vi "Sample To use2.vi"() -> ()   [LabVIEW 2014]
uses:
  Event_class/EventMsg.lvclass
panel:
  in  "Name":string
  out "Msg 3":string
  in  "stop":bool
  in  "Msg 2":string="q2333"
  out "Msg":string
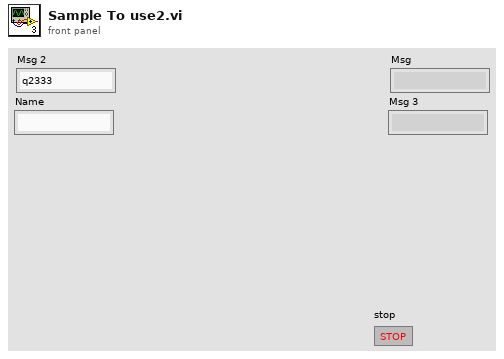
[diagram p1: front panel]
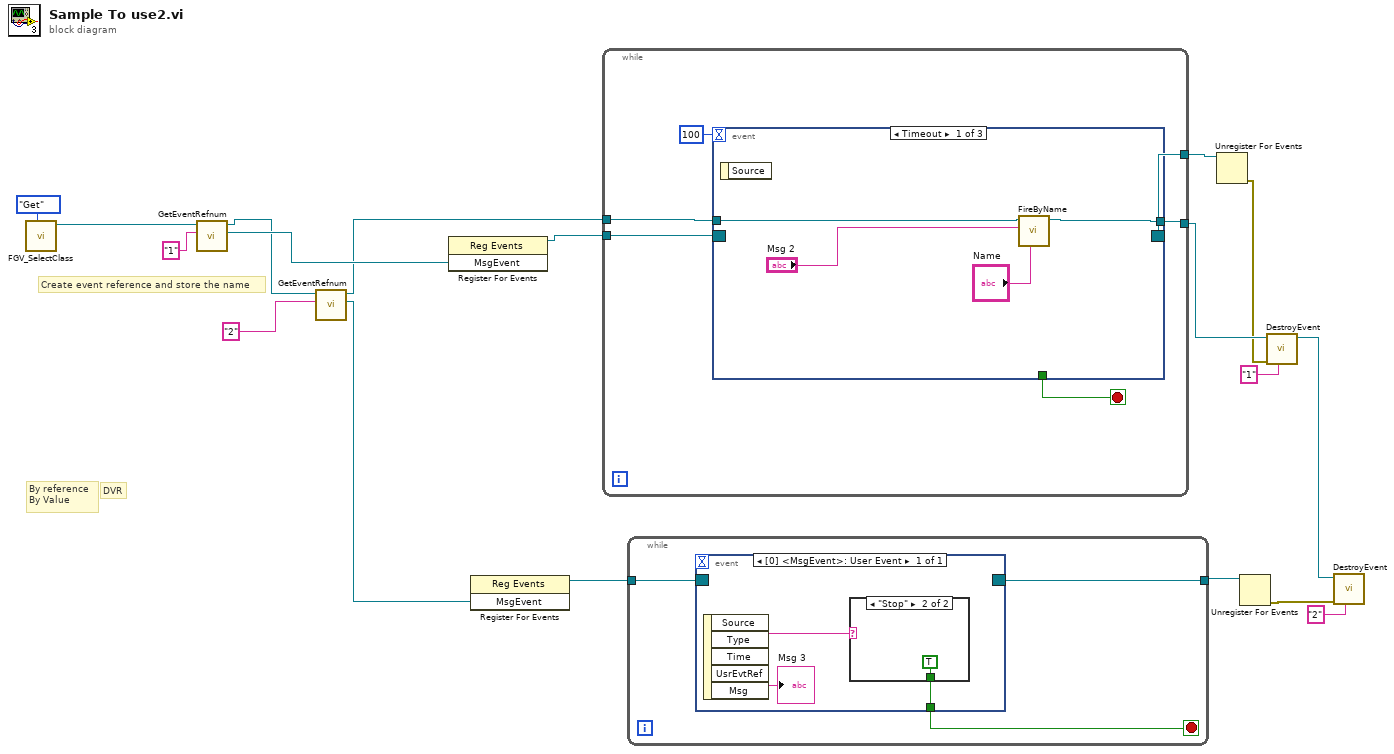
[diagram p0: block diagram]
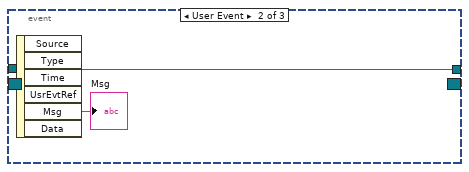
[diagram p3: hidden frame]
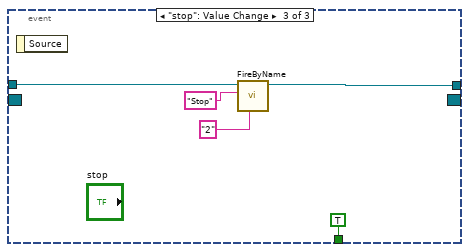
[diagram p4: hidden frame]
diagram:
  # "DVR"
  # "By reference \nBy Value"
  # "Create event reference and store the name"
  n1 = call "FGV_SelectClass.vi"("Action"=enum16{"Set", "Get"}."Get") -> ("EventMsg.lvclass 2"=w1:refnum<class "EventMsg.lvclass">)  [unwired: 10 in]
  n2 = call-dynamic "GetEventRefnum.vi"("Name"="1", "object in"=w1) -> ("MsgEvent"=w8:refnum<user-event>, "object out"=w6:refnum<class "EventMsg.lvclass">)  [unwired: 7 in, 1 out]
  n3 = call-dynamic "GetEventRefnum.vi"("Name"="2", "object in"=w6) -> ("MsgEvent"=w5:refnum<user-event>, "object out"=w3:refnum<class "EventMsg.lvclass">)  [unwired: 7 in, 1 out]
  n4 = register-events(w8) -> (reference out=w18:refnum<event-registration>)  [unwired: 2 in, 1 out]
  n5 = register-events(w5) -> (reference out=w17:refnum<event-registration>)  [unwired: 2 in, 1 out]
  n6 = while {
    tunnel: w18 -> [w23]
    tunnel: w3 -> [w21]
    tunnel: [w20] -> w15
    tunnel: [w19] -> w14
    stop <- w24 stop-if-true
    n7 = event shown="[0] Timeout" {
      selector: w23 -> [_ _ _]
      dyn-events: [_ _ _] -> w19
      timeout: 100 -> [_ _ _]
      tunnel: w21 -> [w27 w29 w33]
      tunnel: [_ _ TRUE ("stop")] -> w24
      tunnel: [w26 w29 w32] -> w20
      event Timeout {
        n8 = event-data() -> ()  [unwired: 1 in, 1 out]
        n9 = call-dynamic "FireByName.vi"("Name"="Name", "Msg"="Msg 2", "object in"=w27) -> ("object out"=w26:refnum<class "EventMsg.lvclass">)  [unwired: 7 in, 1 out]
      }
      event User Event {
        n10 = event-data() -> ("Msg"=→"Msg":string)  [unwired: 1 in, 5 out]
      }
      event "stop": Value Change {
        n11 = event-data() -> ()  [unwired: 1 in, 1 out]
        n12 = call-dynamic "FireByName.vi"("Name"="2", "Msg"="Stop", "object in"=w33) -> ("object out"=w32:refnum<class "EventMsg.lvclass">)  [unwired: 7 in, 1 out]
      }
    }
  }
  n13 = while {
    tunnel: w17 -> [w38]
    tunnel: [w36] -> w16
    stop <- w37 stop-if-true
    n14 = event shown="[0] <MsgEvent>: User Event" {
      selector: w38 -> [_]
      dyn-events: [_] -> w36
      timeout: _ -> [_]
      tunnel: [w39] -> w37
      event User Event {
        n15 = event-data() -> ("Msg"=w40:string)  [unwired: 1 in, 4 out]
        "Msg 3" <- w40
        n16 = case shown="\"Stop\"" w40 {
          tunnel: [_ TRUE] -> w39
          frame "False", Default {
          }
          frame "Stop" {
          }
        }
      }
    }
  }
  n17 = Unregister For Events(event registration refnum=w14) -> (error out=w13:errorcluster)  [unwired: 1 in]
  n18 = Unregister For Events(event registration refnum=w16) -> (error out=w12:errorcluster)  [unwired: 1 in]
  n19 = call-dynamic "DestroyEvent.vi"("Name"="1", "error in (no error)"=w13, "object in"=w15) -> ("object out"=w11:refnum<class "EventMsg.lvclass">)  [unwired: 7 in, 1 out]
  n20 = call-dynamic "DestroyEvent.vi"("Name"="2", "error in (no error)"=w12, "object in"=w11) -> ()  [unwired: 7 in, 2 out]
